vi "Dashboard Main.vi"() -> ()   [LabVIEW 2013]
uses:
  <vilib>/event_ctls.llb/eventvkey.ctl
  <vilib>/Rock Robotics/WPI/Dashboard/WPI_DashboardLogging Global.vi
  <vilib>/Utility/config.llb/Write Key (String).vi
  <vilib>/Utility/config.llb/Write Key (I32).vi
  <vilib>/Utility/config.llb/NI_LVConfig.lvlib
panel:
  out "Image Message":string="Timeout in Camera Communications"
  in  "Rec Mode":enum32{"Stop", "Record", "Playback"}(radio)
  in  "Dashboard Tab":T1(tab)
  in  "Camera Settings":T2={"Frame Rate"=30, "Compression"=30, "Size"=1} {"Frame Rate" scale=1.0..30.0; "Size" items=["640x480", "320x240", "160x120"]}
  out "MotorSliders R":cluster{"MotorSlide1":dbl, "MotorSlide2":dbl} {"MotorSlide2" scale=-1.0..1.0 scale format="%#_2e"; "MotorSlide1" scale=-1.0..1.0 scale format="%#_2e"}
  out "MotorChart R":cluster{"Numeric":dbl, "Numeric":dbl}(graph)
  out "MotorSliders L":T3 {"MotorSlide4 2" scale=0.0..14.0 scale format="%#_2e"; "MotorSlide2" scale=-1.0..1.0 scale format="%#_2e"; "MotorSlide1" scale=-1.0..1.0 scale format="%#_2e"}
  out "MotorChart L":T4(graph)
  out "JS1 Z":dbl(slide) scale=-1.0..1.0 scale format="%#_2e"
  out "Joystick 1":cluster{"X":dbl, "Y":dbl}[](graph)
  out "JS Buttons 1":T5
  out "JS2 Z":dbl(slide) scale=-1.0..1.0 scale format="%#_2e"
  out "Joystick 2":cluster{"X":dbl, "Y":dbl}[](graph)
  out "JS Buttons 2":T5
  out "Mode":T6(ring)=enum."Auto Disabled"
  out "Camera IP":string
  in  "DB Camera Config":bool
  out "fps":dbl format="%#.1g"
  out "Mbps":dbl format="%#.1g"
  out "Mbps 2":bool
  out "LED 1":bool
  in  "Slider 1":dbl(slide) scale=0.0..100.0
  in  "Checkbox 2":bool
  in  "Checkbox 1":bool
  in  "Swag Drive":bool
  out "PID":dbl=3.125
  in  "Set Pot":dbl=3.125
  in  "Smart Shooter":bool=TRUE
  in  "Power Saver":bool=TRUE
  out "Robot Code Version":string
  out "Climber Position":string
  out "Pot Voltage":dbl
  out "Shooter Speed":dbl
  in  "Test Slider":dbl(slide) scale=0.0..100.0 scale format="%#_3g"
  in  "On/Off":bool caption="Solenoid"
  in  "Test Name":u16(ring) items=["Select the test to run...", "Example Test", "-------------------------------", "List of tests is built in robot code.", "Replace with your own automated tests."]
  in  "Test Tree":string(tree)
  in  "Motor":cluster{"Value":dbl, "Enable":bool} {"Value" scale=-1.0..1.0 scale format="%#_3g"}
  out "Progress":T7 {"Test Progress" scale=0.0..100.0}
  in  "Rev/Fwd":cluster{"Forward":bool, "Reverse":bool}
  in  "Test Ring":u16(ring) items=["Auto", "Fixed indoor", "Fixed outdoor 1", "Fixed outdoor 2", "Fixed fluorescent 1", "Fixed fluorescent 2", "Hold current"]
  in  "Listbox":i32(listbox)
  out "Tree":string(tree)
  out "Camera Image":T8(plugin-control)
  in  "Enable":bool
  # "Left"
  # "Front"
  # "Right"
  # "Battery"
  # "Customize by placing controls and indicators here and name to\nmatch Dashboard Variables on robot."
  # "This tab is a great place for autonomous settings and validation.\nCustomize by placing controls and indicators here and name to\nmatch Dashboard Variables on robot."
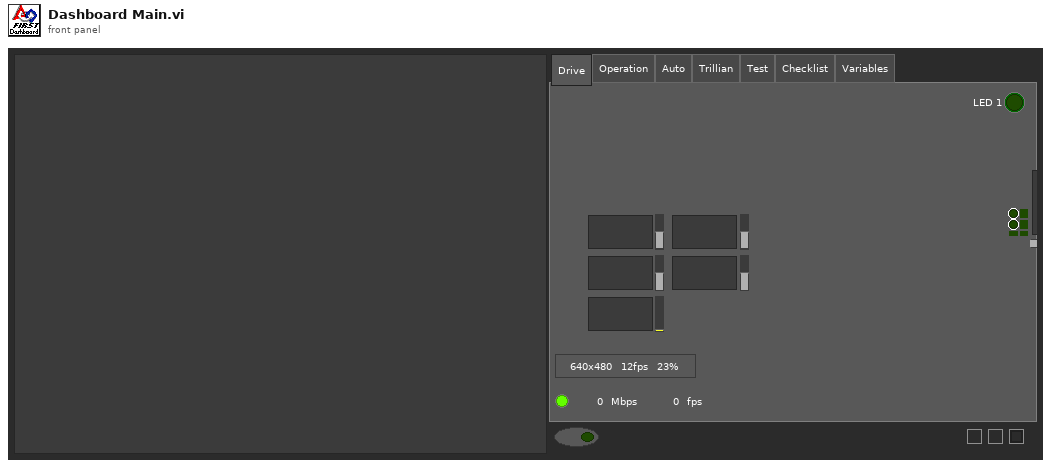
[diagram p1: front panel]
types:
  T1 = enum32{"Drive", "Operation", "Auto", "Trillian", "Test", "Checklist", "Variables"}
  T2 = cluster{"Frame Rate":i32, "Compression":i32, "Size":u16}
  T3 = cluster{"MotorSlide1":dbl, "MotorSlide2":dbl, "MotorSlide4 2":dbl}
  T4 = cluster{"Numeric":dbl, "Numeric":dbl, "Battery":sgl}
  T5 = cluster{bool, bool, bool, bool, bool, bool, bool, bool, bool, bool, bool, bool}
  T6 = enum8{"Tele-Op Disabled", "Tele-Op Enabled", "Auto Disabled", "Auto Enabled", "Test Disabled", "Test Enabled", ""}
  T7 = cluster{"Test Progress":u8, "Test Progress Text":string}
  T8 = typedef "IMAQ Image.ctl" = refnum<image>
  T9 = enum32{"Drive", "Operation", "Auto", "Test", "Checklist", "Variables"}
  T10 = typedef "Image Type" = u32
  T11 = cluster{"Digital Inputs":bool[], "Digital Outputs":bool[]}
  T12 = cluster{"Competition mode":bool, "Robot Link":bool, "Autonomous":bool, "Enabled":bool, "E-Stop":bool, "Simulated":bool, "TestMode":bool, "Docked Window":bool}
  T13 = cluster{"Boolean Array[0]":bool, "Boolean Array[1]":bool, "Boolean Array[2]":bool, "Boolean Array[3]":bool, "Boolean Array[4]":bool, "Boolean Array[5]":bool, "Boolean Array[6]":bool, "Boolean Array[7]":bool, "Boolean Array[8]":bool, "Boolean Array[9]":bool, "Boolean Array[10]":bool, "Boolean Array[11]":bool}
  T14 = typedef "NI_LVConfig.lvlib/Config Data RefNum.ctl" = refnum<k1>
  T15 = typedef "eventvkey.ctl" = enum16{"ASCII", "Enter", "Return", "Shift", "Ctrl", "Alt", "Cmd", "Opt", "Caps", "NumLock", "Clear", "Break", "Up", "Down", "Left", "Right", "Insert", "Delete", "Home", "End", "PageUp", "PageDown", "Escape", "Help", "Pause", "ScrollLock", "F1", "F2", "F3", "F4", "F5", "F6", "F7", "F8", "F9", "F10", "F11", "F12", "F13", "F14", "F15", "F16", "F17", "F18", "F19", "F20", "F21", "F22", "F23", "F24", "Play", "VolumeUp", "VolumeDown", "Mute", "Two Byte Char"}
  T16 = cluster{"Image Size":bool, "Image Type":bool, "Pixel Value":bool, "ROI Information":bool, "Zoom Factor":bool}
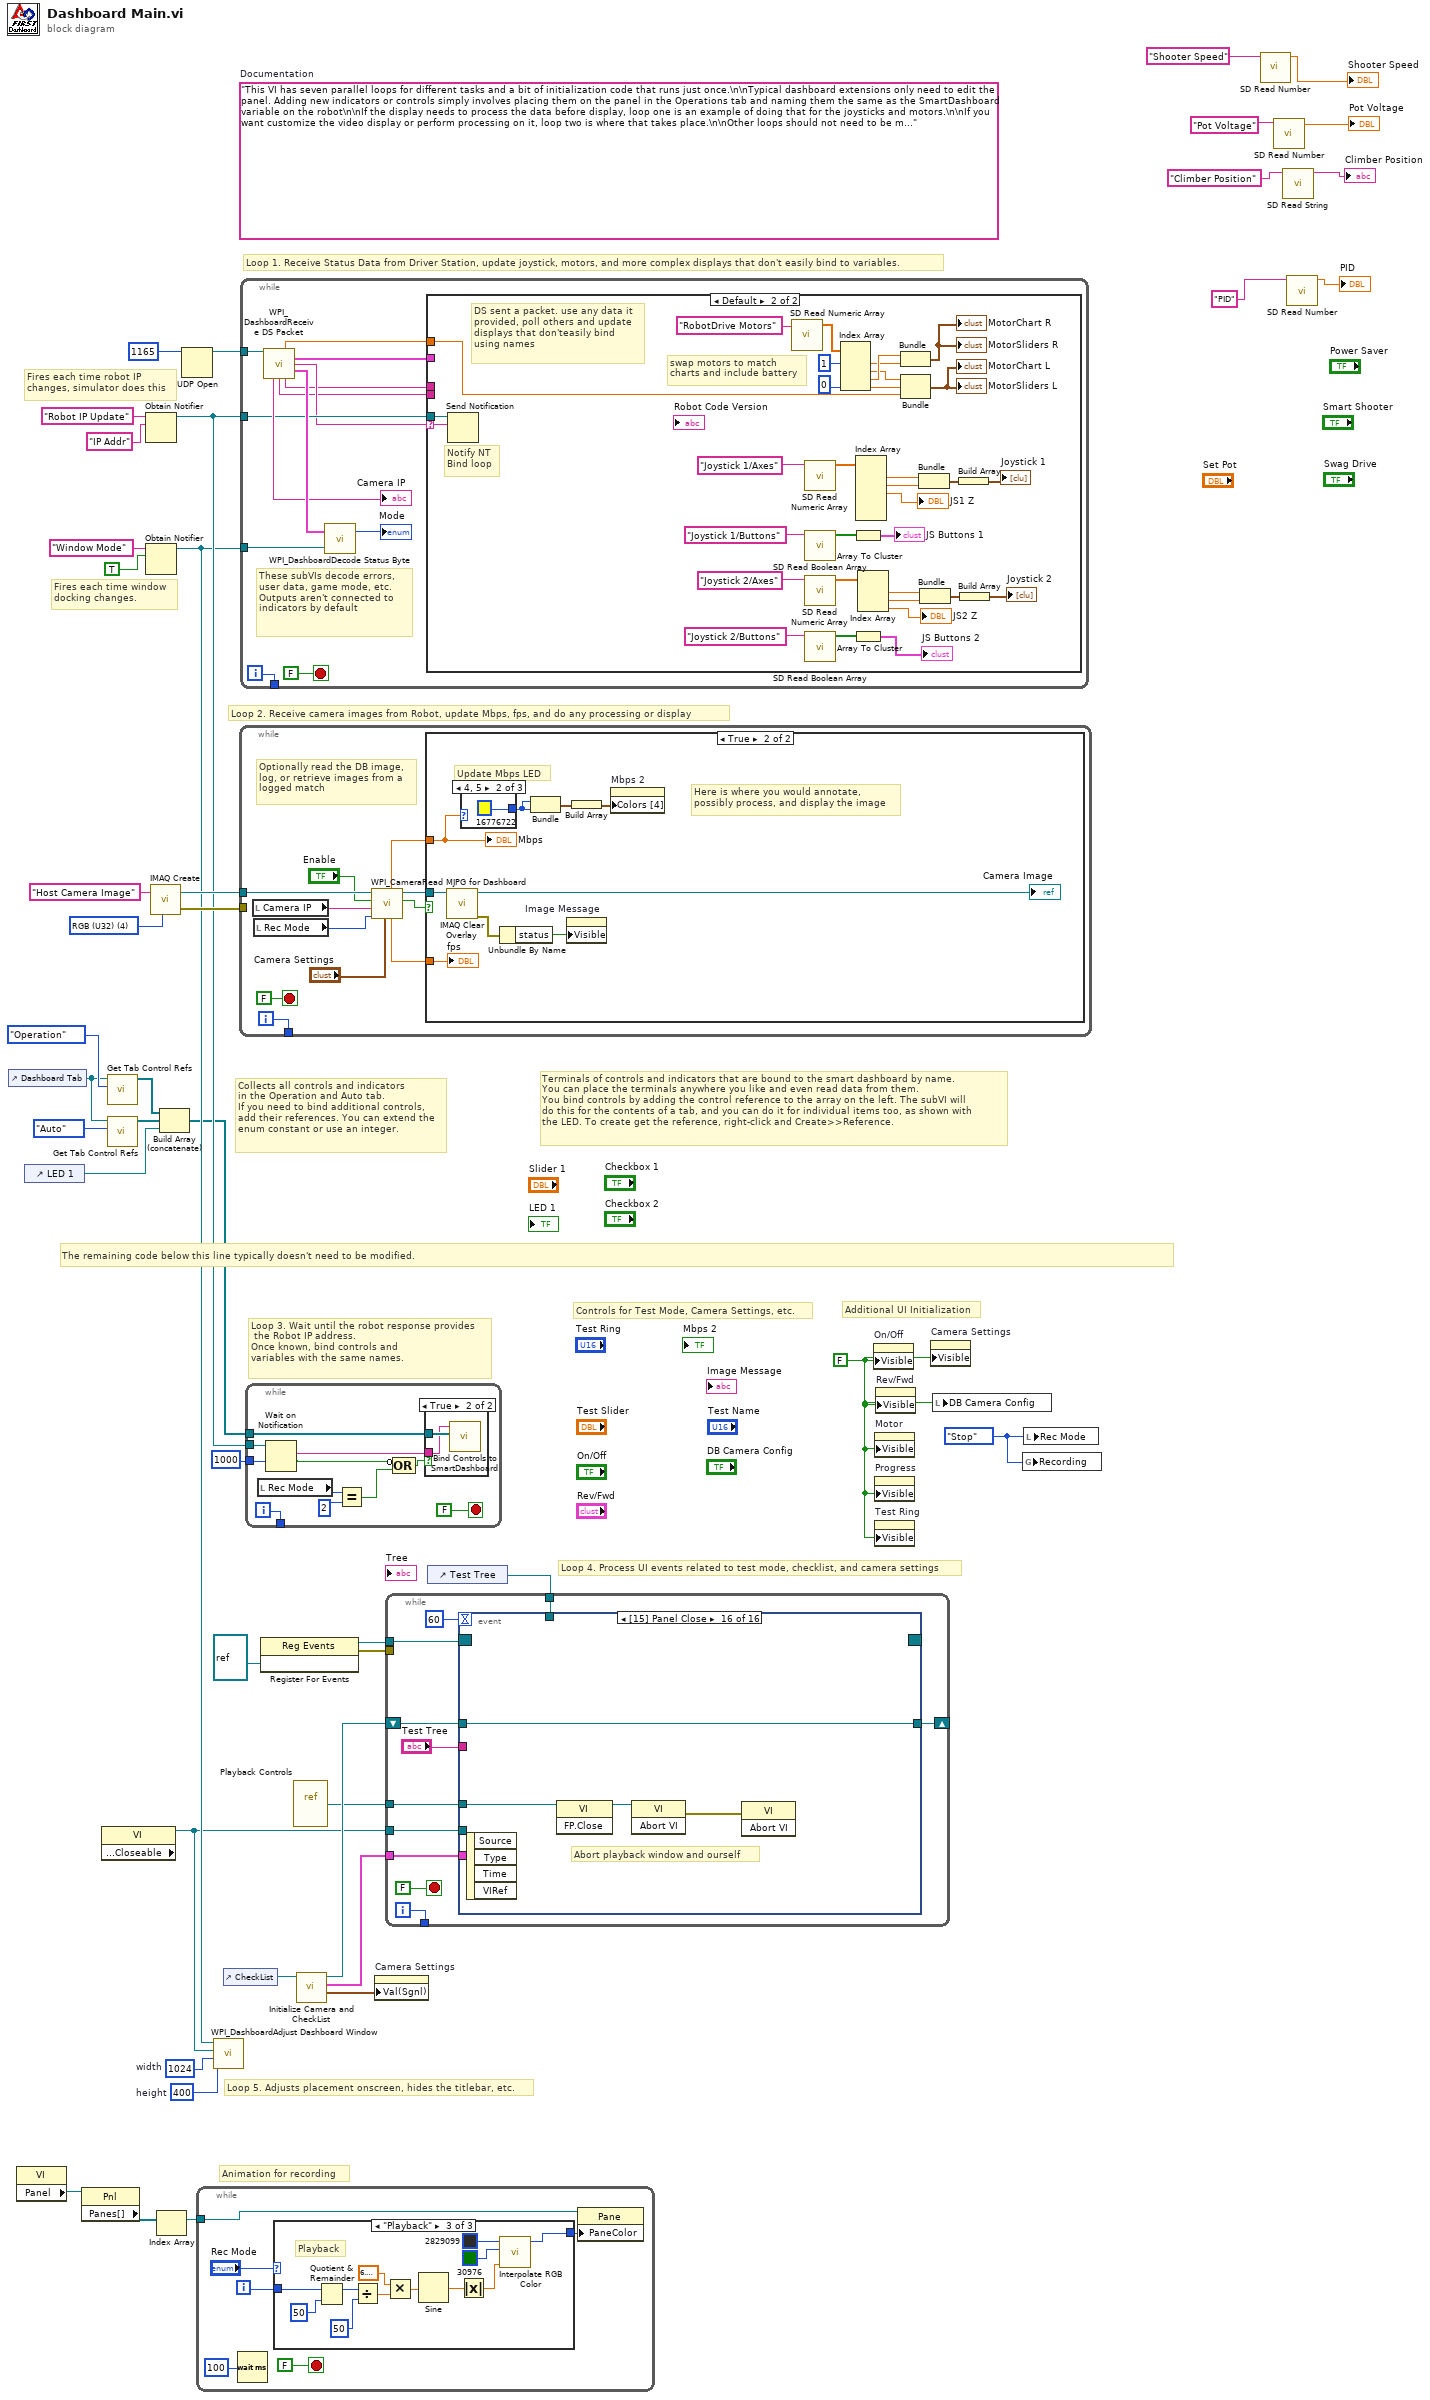
[diagram p0: block diagram]
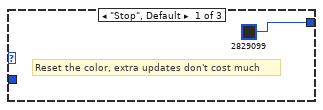
[diagram p2: hidden frame]
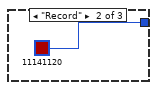
[diagram p3: hidden frame]
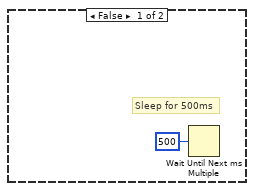
[diagram p5: hidden frame]
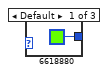
[diagram p6: hidden frame]
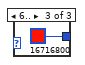
[diagram p7: hidden frame]
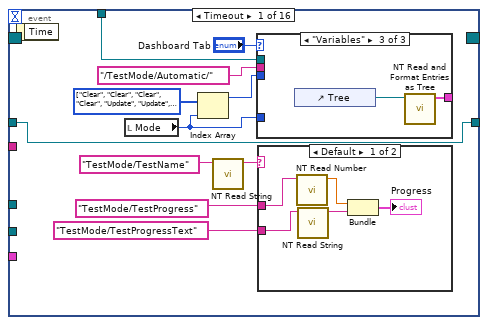
[diagram p8: hidden frame]
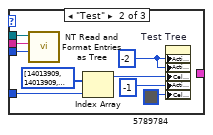
[diagram p10: hidden frame]
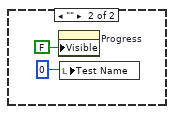
[diagram p11: hidden frame]
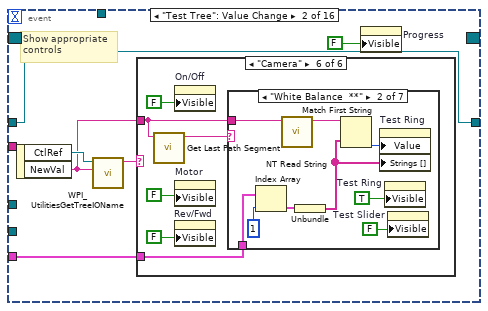
[diagram p12: hidden frame]
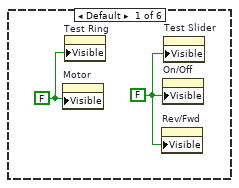
[diagram p13: hidden frame]
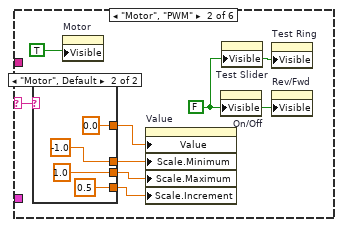
[diagram p14: hidden frame]
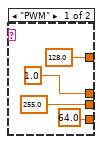
[diagram p15: hidden frame]
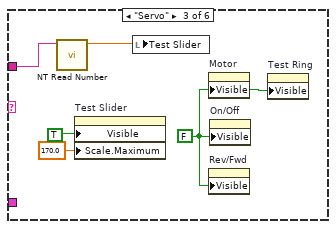
[diagram p16: hidden frame]
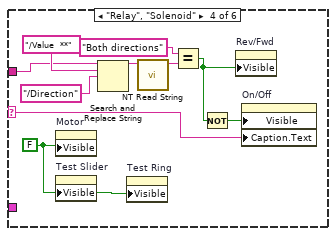
[diagram p17: hidden frame]
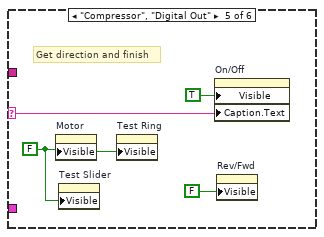
[diagram p18: hidden frame]
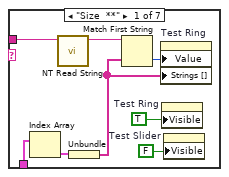
[diagram p19: hidden frame]
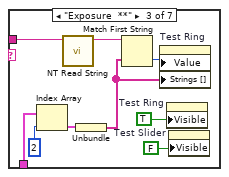
[diagram p20: hidden frame]
diagram:
  w16 = enum32{"Stop", "Record", "Playback"}."Stop" ("Rec Mode")
  w19 = 400  # height
  w20 = 1024  # width
  w33 = FALSE ("Visible")
  (unwired) "This VI has seven parallel loops for different tasks and a bit of initialization code that runs just once.\n\nTypical dashboard extensions only need to edit the panel. Adding new indicators or controls simply involves placing them on the panel in the Operations tab and naming them the same as the SmartDashboard variable on the robot\n\nIf the display needs to process the data before display, loop one is an example of doing that for the joysticks and motors.\n\nIf you want customize the video display or perform processing on it, loop two is where that takes place.\n\nOther loops should not need to be modified. They are pretty standard, and document the task they perform."  # Documentation
  w43 = T10 4 items=["Grayscale (U8)", "Grayscale (I16)", "Grayscale (SGL)", "Complex (CSG)", "RGB (U32)", "HSL (U32)", "RGB (U64)"] ("Image Type")
  # "Controls for Test Mode, Camera Settings, etc."
  # "Additional UI Initialization"
  # "Animation for recording"
  # "Fires each time robot IP\nchanges, simulator does this"
  # "Fires each time window\ndocking changes."
  # "Collects all controls and indicators\nin the Operation and Auto tab.\nIf you need to bind additional controls,\nadd their references. You can extend the\nenum constant or use an integer."
  # "The remaining code below this line typically doesn't need to be modified."
  # "Loop 4. Process UI events related to test mode, checklist, and camera settings"
  # "Terminals of controls and indicators that are bound to the smart dashboard by name.\nYou can place the terminals anywhere you like and even read data from them.\nYou bind controls by adding the control reference to the array on the left. The subVI will\ndo this for the contents of a tab, and you can do it for individual items too, as shown with\nthe LED. To create get the reference, right-click and Create>>Reference."
  # "Loop 3. Wait until the robot response provides\n the Robot IP address.\nOnce known, bind controls and\nvariables with the same names."
  # "Loop 5. Adjusts placement onscreen, hides the titlebar, etc."
  # "Loop 1. Receive Status Data from Driver Station, update joystick, motors, and more complex displays that don't easily bind to variables."
  # "Loop 2. Receive camera images from Robot, update Mbps, fps, and do any processing or display"
  n1 = control-ref of="Dashboard Tab"() -> (w14:refnum<vi>)
  n2 = property class="VI"() -> ("Panel"=w27:refnum<vi>)  [unwired: 2 in, 2 out]
  n3 = control-ref of="LED 1"() -> (w9:refnum<vi>)
  n4 = property class="Pnl"(reference=w27) -> ("Panes[]"=w28:refnum<vi>[])  [unwired: 1 in, 2 out]
  n5 = property class="VI" props=["Front Panel.Closeable"]() -> (reference out=w15:refnum<vi>)  [unwired: 2 in, 2 out]
  n6 = call <vilib>:"Get Tab Control Refs.vi"("Page Index"=T9."Operation" ("Dashboard Tab"), "TabControl in"=w14) -> ("ControlsOnPage"=w12:refnum<vi>[])  [unwired: 9 in]
  n7 = call <vilib>:"Get Tab Control Refs.vi"("Page Index"=T9."Auto" ("Dashboard Tab"), "TabControl in"=w14) -> ("ControlsOnPage"=w13:refnum<vi>[])  [unwired: 9 in]
  n8 = Obtain Notifier(name (unnamed)="Robot IP Update", notification data type="IP Addr" ("name (unnamed)")) -> (notifier out=w37:refnum<notifier>)  [unwired: 2 in, 2 out]
  n9 = Obtain Notifier(name (unnamed)="Window Mode", notification data type=TRUE) -> (notifier out=w18:refnum<notifier>)  [unwired: 2 in, 2 out]
  n10 = call "IMAQ Create"("Image Name"="Host Camera Image", "Image Type"=w43) -> ("New Image"=w41:T8, "error out"=w40:errorcluster)  [unwired: 2 in, 1 out]
  n11 = Index Array(array=w28) -> (element=w26:refnum<vi>)  [unwired: 1 in]
  n12 = Build Array (concatenate)(w12, w13, w9) -> (w11:refnum<vi>[])
  n13 = UDP Open(11:u16 1165 ("port")) -> (port=w44:refnum<k16>)  [unwired: 2 in, 4 out]
  n14 = while {
    tunnel: w26 -> [w47]
    i -> [w50]
    stop <- FALSE stop-if-true
    n15 = Wait (ms)(milliseconds to wait=u32 100) -> ()  [unwired: 1 out]
    n16 = case shown="\"Playback\"" "Rec Mode" {
      tunnel: w50 -> [_ _ w65]
      tunnel: [u32 2829099 ("Base Color") u32 11141120 ("Target Color") w54] -> w46
      frame "Stop", Default {
        # "Reset the color, extra updates don't cost much"
      }
      frame "Record" {
      }
      frame "Playback" {
        # "Playback"
        n17 = Quotient & Remainder(x=w65, y=u32 50 ("milliseconds to wait")) -> (x-y*floor(x/y)=w61:u32)  [unwired: 1 out]
        n18 = Divide(x=w61, y=u32 50 ("milliseconds to wait")) -> (x/y=w58:dbl)
        n19 = Multiply(x=6.283185307179586, y=w58) -> (x*y=w63:dbl)
        n20 = Sine(x=w63) -> (sin(x)=w62:dbl)
        n21 = Absolute Value(x=w62) -> (abs(x)=w55:dbl)
        n22 = call "Interpolate RGB Color.vi"("Proportion"=w55, "Target Color"=u32 30976, "Base Color"=u32 2829099) -> ("Result Color"=w54:u32)  [unwired: 8 in]
      }
    }
    n23 = property class="Pane"(reference=w47, "PaneColor"=w46) -> ()  [unwired: 1 in, 2 out]
  }
  n24 = call <vilib>:"WPI_DashboardAdjust Dashboard Window.vi"("height"=w19, "width"=w20, "reference in"=w15, "Notifier in"=w18) -> ()  [unwired: 8 in]
  n25 = control-ref of="CheckList"() -> (w17:refnum<vi>)
  n26 = while {
    tunnel: w41 -> [w74]
    tunnel: w40 -> [_]
    tunnel: [w75] -> _
    i -> [w75]
    stop <- FALSE stop-if-true
    # "Optionally read the DB image,\nlog, or retrieve images from a\nlogged match"
    n27 = local read "Camera IP"() -> (w67:string)
    n28 = local read "Rec Mode"() -> (w66:enum32{"Stop", "Record", "Playback"})
    n29 = call <vilib>:"WPI_CameraRead MJPG for Dashboard.vi"("Camera Settings"="Camera Settings", "Rec Mode"=w66, "Camera IP"=w67, "Enable"="Enable", "Refnum in"=w74) -> ("Active"=w71:bool, "Refnum out"=w73:T8, "FPS"=w70:dbl, "Bandwidth (Mbps)"=w69:dbl)  [unwired: 3 in]
    n30 = case shown="True" w71 {
      tunnel: w73 -> [_ w81]
      tunnel: w69 -> [_ w80]
      tunnel: w70 -> [_ w78]
      frame False {
        # "Sleep for 500ms"
        n31 = Wait Until Next ms Multiple(millisecond multiple=u32 500) -> ()  [unwired: 1 out]
      }
      frame True {
        # "Here is where you would annotate,\npossibly process, and display the image"
        # "Update Mbps LED"
        n32 = call "IMAQ Clear Overlay"("Image"=w81) -> ("error out"=w85:errorcluster, "Image Out"=→"Camera Image":T8)  [unwired: 2 in, 7 out]
        n33 = case shown="4, 5" w80 {
          tunnel: [u32 6618880 ("Color Box") u32 16776722 ("Color Box") u32 16716800 ("Color Box")] -> w82
          frame Default {
          }
          frame 4, 5 {
          }
          frame 6.. {
          }
        }
        n34 = Unbundle By Name(w85) -> ("status"=w86:bool)
        n35 = Bundle("Color Box"=w82, "Color Box"=w82) -> (w84:cluster{"Color Box":u32, "Color Box":u32})  [unwired: 1 out]
        n36 = property on="Image Message" class="Str"("Visible"=w86) -> ()  [unwired: 2 in, 2 out]
        n37 = Build Array(w84) -> (w83:cluster{"Color Box":u32, "Color Box":u32}[])
        n38 = property on="Mbps 2" class="Bool (strict)"("Colors [4]"=w83) -> ()  [unwired: 2 in, 2 out]
        "Mbps" <- w80
        "fps" <- w78
      }
    }
  }
  n39 = while {
    tunnel: w44 -> [w100]
    tunnel: w37 -> [w95]
    tunnel: w18 -> [w99]
    tunnel: [w96] -> _
    i -> [w96]
    stop <- FALSE stop-if-true
    # "These subVIs decode errors, user data, game mode, etc.\nOutputs aren't connected to indicators by default"
    n40 = call <vilib>:"WPI_DashboardReceive DS Packet.vi"("Recv Socket"=w100) -> ("Battery"=w90:sgl, "Driver Station"=w91:T11, "Robot IP Address"=w94:string, "Status"=w101:T12, "Camera IP Address"=→"Camera IP":string, "Low Priority User Data"=w93:string, "High Priority User Data"=w92:string)  [unwired: 1 in, 7 out]
    n41 = call <vilib>:"WPI_DashboardDecode Status Byte.vi"("Window Mode Notifier"=w99, "Status"=w101) -> ("Mode"=→"Mode":T6)  [unwired: 1 out]
    n42 = case shown="Default" w94 {
      selector: w94 -> [_ w113]
      tunnel: w95 -> [_ w114]
      tunnel: w93 -> [_ _]
      tunnel: w92 -> [_ _]
      tunnel: w91 -> [_ _]
      tunnel: w90 -> [_ w112]
      frame "0.0.0.0" {
        # "DS not sending packets, or no robot exists yet.\nDon't poll the variables"
      }
      frame Default {
        # "Notify NT\nBind loop"
        # "DS sent a packet. use any data it\nprovided, poll others and update\ndisplays that don'teasily bind\nusing names"
        # "swap motors to match\ncharts and include battery"
        n43 = Send Notification(notification=w113, notifier=w114) -> ()  [unwired: 1 in, 2 out]
        n44 = call <vilib>:"SD Read Numeric Array.vi"("Name"="RobotDrive Motors") -> ("Numeric Array"=w111:dbl[])  [unwired: 8 in, 2 out]
        n45 = call <vilib>:"SD Read Numeric Array.vi"("Name"="Joystick 1/Axes") -> ("Numeric Array"=w130:dbl[])  [unwired: 8 in, 2 out]
        n46 = call <vilib>:"SD Read Boolean Array.vi"("Name"="Joystick 1/Buttons") -> ("Boolean Array"=w132:bool[])  [unwired: 8 in, 2 out]
        n47 = call <vilib>:"SD Read Numeric Array.vi"("Name"="Joystick 2/Axes") -> ("Numeric Array"=w124:dbl[])  [unwired: 8 in, 2 out]
        n48 = call <vilib>:"SD Read Boolean Array.vi"("Name"="Joystick 2/Buttons") -> ("Boolean Array"=w123:bool[])  [unwired: 8 in, 2 out]
        n49 = Index Array(array=w111, index #1=1, index #4=0) -> (element #1=w107:dbl, element #2=w106:dbl, element #3=w108:dbl, element #4=w103:dbl)  [unwired: 2 in]
        n50 = Array To Cluster(array=w132) -> (cluster=→"JS Buttons 1":T13)
        n51 = Array To Cluster(array=w123) -> (cluster=→"JS Buttons 2":T13)
        n52 = Index Array(array=w130) -> (element #1=w127:dbl, element #2=w128:dbl, element #3=→"JS1 Z":dbl)  [unwired: 6 in, 3 out]
        n53 = Index Array(array=w124) -> (element #1=w119:dbl, element #2=w118:dbl, element #3=→"JS2 Z":dbl)  [unwired: 3 in]
        n54 = Bundle("Numeric"=w108, "Numeric"=w107) -> (→"MotorChart R" →"MotorSliders R":cluster{"Numeric":dbl, "Numeric":dbl})  [unwired: 1 in]
        n55 = Bundle("Numeric"=w106, "Numeric"=w103, "Battery"=w112) -> (→"MotorChart L" →"MotorSliders L":T4)  [unwired: 1 in]
        n56 = Bundle("Numeric"=w127, "Numeric"=w128) -> (w126:cluster{"Numeric":dbl, "Numeric":dbl})  [unwired: 1 in]
        n57 = Bundle("Numeric"=w119, "Numeric"=w118) -> (w120:cluster{"Numeric":dbl, "Numeric":dbl})  [unwired: 1 in]
        n58 = Build Array(w126) -> (→"Joystick 1":cluster{"Numeric":dbl, "Numeric":dbl}[])
        n59 = Build Array(w120) -> (→"Joystick 2":cluster{"Numeric":dbl, "Numeric":dbl}[])
      }
    }
  }
  n60 = while {
    tunnel: w11 -> [w146]
    tunnel: w37 -> [w144]
    tunnel: [w142] -> _
    tunnel: u32 1000 ("milliseconds to wait") -> [w141]
    i -> [w142]
    stop <- FALSE stop-if-true
    n61 = local read "Rec Mode"() -> (w137:enum32{"Stop", "Record", "Playback"})
    n62 = Wait on Notification(notifier=w144, timeout in ms (-1)=w141) -> (notification=w143:string, timed out?=w139:bool)  [unwired: 2 in, 2 out]
    n63 = Equal?(x=w137, y=u16 2 ("Rec Mode")) -> (x = y?=w138:bool)
    n64 = Compound Arithmetic op=OR(invert w139, w138) -> (w140:bool)
    n65 = case shown="True" w140 {
      tunnel: w146 -> [_ w148]
      tunnel: w143 -> [_ w147]
      frame False {
      }
      frame True {
        n66 = call <vilib>:"Bind Controls to SmartDashboard.vi"("Bound Control Refs"=w148, "Server IP Address"=w147) -> ()  [unwired: 10 in]
      }
    }
  }
  n67 = register-events(refnum<vi> refnum) -> (reference out=w24:refnum<event-registration>, error out=w23:errorcluster)  [unwired: 2 in]
  n68 = vi-ref "Playback Controls.vi"() -> (w25:refnum<vi>)
  n69 = call "Initialize Camera and CheckList.vi"("ListBox in"=w17) -> ("Cluster"=w31:cluster{"value":i32, "value":i32, "index":i32}, "Array"=w32:cluster{string[]}[], "File Refnum"=w30:T14)  [unwired: 8 in]
  n70 = property on="Camera Settings" class="Clust (strict)"("Val(Sgnl)"=w31) -> ()  [unwired: 2 in, 2 out]
  n71 = control-ref of="Test Tree"() -> (w29:refnum<vi>)
  n72 = while {
    tunnel: w32 -> [w156]
    shift-right: [w155] -> _
    shift-left: w30 -> [w154]
    tunnel: [w153] -> _
    tunnel: w29 -> [w152]
    tunnel: w25 -> [w151]
    tunnel: w24 -> [w150]
    tunnel: w23 -> [_]
    tunnel: w15 -> [w149]
    i -> [w153]
    stop <- FALSE stop-if-true
    n73 = event shown="[15] Panel Close" {
      selector: w150 -> [_ _ _ _ _ _ _ _ _ _ _ _ _ _ _ _]
      dyn-events: [_ _ _ _ _ _ _ _ _ _ _ _ _ w394 _ _] -> _
      timeout: u32 60 ("milliseconds to wait") -> [_ _ _ _ _ _ _ _ _ _ _ _ _ _ _ _]
      tunnel: w152 -> [w166 _ _ _ _ _ _ _ _ _ _ _ _ _ _ _]
      tunnel: "Test Tree" -> [_ _ _ _ _ _ _ _ w363 w371 w373 w377 w385 _ _ _]
      tunnel: w156 -> [_ w190 _ _ _ _ w327 w357 _ _ _ _ _ _ _ _]
      tunnel: [w160 w189 w288 w293 w301 w313 w326 w350 w362 w369 w372 w376 w384 w396 w410 w411] -> w155
      tunnel: w154 -> [w160 w189 w288 w293 w301 w313 w325 w350 w362 w369 w372 w376 w384 w396 w410 w411]
      tunnel: w151 -> [_ _ _ _ _ _ _ _ _ _ _ _ _ w397 _ w414]
      tunnel: w149 -> [_ _ _ _ _ _ _ _ _ _ _ _ _ w392 _ _]
      event Timeout {
        w165 = enum16{"Update", "Clear"}[] [enum."Clear", enum."Clear", enum."Clear", enum."Clear", enum."Update", enum."Update", enum."Clear"] items=["Update", "Clear"]
        n74 = event-data() -> ()  [unwired: 1 in, 1 out]
        n75 = local read "Mode"() -> (w163:T6)
        n76 = Index Array(array=w165, index=w163) -> (element=w164:enum16{"Update", "Clear"})
        n77 = call <vilib>:"NT Read String.vi"("Name"="TestMode/TestName") -> ("String"=w169:string)  [unwired: 9 in, 1 out]
        n78 = case shown="\"Variables\"" "Dashboard Tab" {
          tunnel: w166 -> [_ w179 _]
          tunnel: "/TestMode/Automatic/" ("Name Pattern") -> [_ w178 _]
          tunnel: w164 -> [_ w177 _]
          tunnel: w163 -> [_ w175 _]
          tunnel: [_ _ w181] -> _
          frame "Operation", Default {
          }
          frame "Test" {
            w174 = -2 ("Active Item:Row Number")
            n79 = call <vilib>:"NT Read and Format Entries as Tree.vi"("Operation"=w177, "Name Pattern"=w178, "Tree Refnum"=w179) -> ()  [unwired: 7 in, 2 out]
            n80 = Index Array(array=u32[] [14013909, 14013909, 14013909, 14013909, 14013909, 16777215, 14013909], index=w175) -> (element=w173:u32)
            n81 = property on="Test Tree" class="Tree (strict)"("Active Item Row Number"=w174, "ActiveColNum"=w174, "CellBG"=w173, "Active Item Row Number"=-1 ("Active Item:Row Number"), "CellBG"=u32 5789784 ("Color Box")) -> ()  [unwired: 2 in, 2 out]
          }
          frame "Variables" {
            n82 = control-ref of="Tree"() -> (w180:refnum<vi>)
            n83 = call <vilib>:"NT Read and Format Entries as Tree.vi"("Tree Refnum"=w180) -> ("Formatted Strings"=w181:cluster{"Name":string, "Value":string}[])  [unwired: 9 in, 1 out]
          }
        }
        n84 = case shown="Default" w169 {
          tunnel: "TestMode/TestProgress" ("Name") -> [w183 _]
          tunnel: "TestMode/TestProgressText" ("Name") -> [w182 _]
          frame Default {
            n85 = call <vilib>:"NT Read Number.vi"("Name"=w183) -> ("Numeric"=w184:dbl)  [unwired: 9 in, 1 out]
            n86 = call <vilib>:"NT Read String.vi"("Name"=w182) -> ("String"=w185:string)  [unwired: 9 in, 1 out]
            n87 = Bundle("Numeric"=w184, "String"=w185) -> (→"Progress":cluster{"Numeric":dbl, "String":string})  [unwired: 1 in]
          }
          frame "" {
            n88 = property on="Progress" class="Clust (strict)"("Visible"=FALSE) -> ()  [unwired: 2 in, 2 out]
            n89 = local write "Test Name"(u16 0) -> ()
          }
        }
      }
      event "Test Tree": Value Change {
        # "Show appropriate\ncontrols"
        n90 = event-data() -> ("CtlRef"=w193:refnum<vi>, "NewVal"=w191:string)  [unwired: 1 in]
        n91 = call <vilib>:"WPI_UtilitiesGetTreeIOName.vi"("NewVal"=w191, "TreeControl in"=w193) -> ("I/O Name"=w194:string)  [unwired: 9 in]
        n92 = case shown="\"Camera\"" w194 {
          selector: w194 -> [_ w201 _ w219 w228 _]
          tunnel: w191 -> [_ _ w216 w218 _ w235]
          tunnel: w190 -> [_ _ _ _ _ w234]
          frame Default {
            w196 = FALSE ("Visible")
            w195 = FALSE ("Visible")
            n93 = property on="Motor" class="Clust (strict)"("Visible"=w195) -> ()  [unwired: 2 in, 2 out]
            n94 = property on="Test Ring" class="Ring (strict)"("Visible"=w195) -> ()  [unwired: 2 in, 2 out]
            n95 = property on="Rev/Fwd" class="Clust (strict)"("Visible"=w196) -> ()  [unwired: 2 in, 2 out]
            n96 = property on="On/Off" class="Bool (strict)"("Visible"=w196) -> ()  [unwired: 2 in, 2 out]
            n97 = property on="Test Slider" class="Slide (strict)"("Visible"=w196) -> ()  [unwired: 2 in, 2 out]
          }
          frame "Motor", "PWM" {
            w202 = FALSE ("Visible")
            n98 = case shown="\"Motor\", Default" w201 {
              tunnel: [1.0 ("Value") -1.0 ("Value")] -> w200
              tunnel: [255.0 ("Value") 1.0 ("Value")] -> w199
              tunnel: [128.0 ("Value") 0.0 ("Value")] -> w198
              tunnel: [64.0 ("Value") 0.5 ("Value")] -> w197
              frame "PWM" {
              }
              frame "Motor", Default {
              }
            }
            n99 = property on="Motor" class="Clust (strict)"("Visible"=TRUE) -> ()  [unwired: 2 in, 2 out]
            n100 = property on="Value" class="Slide (strict)"("Value"=w198, "Scale.Minimum"=w200, "Scale.Maximum"=w199, "Scale.Increment"=w197) -> ()  [unwired: 2 in, 2 out]
            n101 = property on="On/Off" class="Bool (strict)"("Visible"=w202) -> ()  [unwired: 2 in, 2 out]
            n102 = property on="Test Slider" class="Slide (strict)"("Visible"=w202) -> ()  [unwired: 2 in, 2 out]
            n103 = property on="Test Ring" class="Ring (strict)"("Visible"=w202) -> ()  [unwired: 2 in, 2 out]
            n104 = property on="Rev/Fwd" class="Clust (strict)"("Visible"=w202) -> ()  [unwired: 2 in, 2 out]
          }
          frame "Servo" {
            w214 = FALSE ("Visible")
            n105 = call <vilib>:"NT Read Number.vi"("Name"=w216) -> ("Numeric"=w215:dbl)  [unwired: 9 in, 1 out]
            n106 = property on="Test Slider" class="Slide (strict)"("Visible"=TRUE, "Scale.Maximum"=170.0 ("Scale.Range:Maximum")) -> ()  [unwired: 2 in, 2 out]
            n107 = local write "Test Slider"(w215) -> ()
            n108 = property on="Motor" class="Clust (strict)"("Visible"=w214) -> ()  [unwired: 2 in, 2 out]
            n109 = property on="Rev/Fwd" class="Clust (strict)"("Visible"=w214) -> ()  [unwired: 2 in, 2 out]
            n110 = property on="On/Off" class="Bool (strict)"("Visible"=w214) -> ()  [unwired: 2 in, 2 out]
            n111 = property on="Test Ring" class="Ring (strict)"("Visible"=w214) -> ()  [unwired: 2 in, 2 out]
          }
          frame "Relay", "Solenoid" {
            w217 = FALSE ("Visible")
            n112 = property on="Motor" class="Clust (strict)"("Visible"=w217) -> ()  [unwired: 2 in, 2 out]
            n113 = property on="Test Slider" class="Slide (strict)"("Visible"=w217) -> ()  [unwired: 2 in, 2 out]
            n114 = Search and Replace String(input string=w218, search string="/Value  **", replace string="/Direction") -> (result string=w224:string)  [unwired: 5 in, 3 out]
            n115 = property on="Test Ring" class="Ring (strict)"("Visible"=w217) -> ()  [unwired: 2 in, 2 out]
            n116 = call <vilib>:"NT Read String.vi"("Name"=w224) -> ("String"=w222:string)  [unwired: 9 in, 1 out]
            n117 = Equal?(x="Both directions", y=w222) -> (x = y?=w220:bool)
            n118 = Not(x=w220) -> (.not. x?=w221:bool)
            n119 = property on="Rev/Fwd" class="Clust (strict)"("Visible"=w220) -> ()  [unwired: 2 in, 2 out]
            n120 = property on="On/Off" class="Bool (strict)"("Visible"=w221, "Caption.Text"=w219) -> ()  [unwired: 2 in, 2 out]
          }
          frame "Compressor", "Digital Out" {
            w227 = FALSE ("Visible")
            # "Get direction and finish"
            n121 = property on="Motor" class="Clust (strict)"("Visible"=w227) -> ()  [unwired: 2 in, 2 out]
            n122 = property on="Test Slider" class="Slide (strict)"("Visible"=w227) -> ()  [unwired: 2 in, 2 out]
            n123 = property on="Test Ring" class="Ring (strict)"("Visible"=w227) -> ()  [unwired: 2 in, 2 out]
            n124 = property on="On/Off" class="Bool (strict)"("Visible"=TRUE, "Caption.Text"=w228) -> ()  [unwired: 2 in, 2 out]
            n125 = property on="Rev/Fwd" class="Clust (strict)"("Visible"=FALSE) -> ()  [unwired: 2 in, 2 out]
          }
          frame "Camera" {
            n126 = call <vilib>:"Get Last Path Segment.vi"("String in"=w235) -> ("String out"=w236:string)  [unwired: 10 in]
            n127 = property on="On/Off" class="Bool (strict)"("Visible"=FALSE) -> ()  [unwired: 2 in, 2 out]
            n128 = property on="Motor" class="Clust (strict)"("Visible"=FALSE) -> ()  [unwired: 2 in, 2 out]
            n129 = property on="Rev/Fwd" class="Clust (strict)"("Visible"=FALSE) -> ()  [unwired: 2 in, 2 out]
            n130 = case shown="\"White Balance  **\"" w236 {
              tunnel: w235 -> [w242 w251 w260 w269 w278 _ w284]
              tunnel: w234 -> [w240 w248 w257 w266 w275 _ _]
              frame "Size  **" {
                n131 = Index Array(array=w240) -> (element=w239:cluster{string[]})  [unwired: 1 in]
                n132 = call <vilib>:"NT Read String.vi"("Name"=w242) -> ("String"=w241:string)  [unwired: 9 in, 1 out]
                n133 = Unbundle(w239) -> (w237:string[])
                n134 = Match First String(2:w237, 3:w241) -> (0:w238:i32)  [unwired: 1 out]
                n135 = property on="Test Ring" class="Ring (strict)"("Value"=w238, "Strings []"=w237) -> ()  [unwired: 2 in, 2 out]
                n136 = property on="Test Ring" class="Ring (strict)"("Visible"=TRUE) -> ()  [unwired: 2 in, 2 out]
                n137 = property on="Test Slider" class="Slide (strict)"("Visible"=FALSE) -> ()  [unwired: 2 in, 2 out]
              }
              frame "White Balance  **" {
                n138 = Index Array(array=w248, index=1) -> (element=w249:cluster{string[]})
                n139 = call <vilib>:"NT Read String.vi"("Name"=w251) -> ("String"=w250:string)  [unwired: 9 in, 1 out]
                n140 = Unbundle(w249) -> (w246:string[])
                n141 = Match First String(2:w246, 3:w250) -> (0:w245:i32)  [unwired: 1 out]
                n142 = property on="Test Ring" class="Ring (strict)"("Value"=w245, "Strings []"=w246) -> ()  [unwired: 2 in, 2 out]
                n143 = property on="Test Ring" class="Ring (strict)"("Visible"=TRUE) -> ()  [unwired: 2 in, 2 out]
                n144 = property on="Test Slider" class="Slide (strict)"("Visible"=FALSE) -> ()  [unwired: 2 in, 2 out]
              }
              frame "Exposure  **" {
                n145 = Index Array(array=w257, index=2) -> (element=w258:cluster{string[]})
                n146 = call <vilib>:"NT Read String.vi"("Name"=w260) -> ("String"=w259:string)  [unwired: 9 in, 1 out]
                n147 = Unbundle(w258) -> (w254:string[])
                n148 = Match First String(2:w254, 3:w259) -> (0:w255:i32)  [unwired: 1 out]
                n149 = property on="Test Ring" class="Ring (strict)"("Value"=w255, "Strings []"=w254) -> ()  [unwired: 2 in, 2 out]
                n150 = property on="Test Ring" class="Ring (strict)"("Visible"=TRUE) -> ()  [unwired: 2 in, 2 out]
                n151 = property on="Test Slider" class="Slide (strict)"("Visible"=FALSE) -> ()  [unwired: 2 in, 2 out]
              }
              frame "Exposure Priority  **" {
                n152 = Index Array(array=w266, index=3) -> (element=w267:cluster{string[]})
                n153 = call <vilib>:"NT Read String.vi"("Name"=w269) -> ("String"=w268:string)  [unwired: 9 in, 1 out]
                n154 = Unbundle(w267) -> (w263:string[])
                n155 = Match First String(2:w263, 3:w268) -> (0:w264:i32)  [unwired: 1 out]
                n156 = property on="Test Ring" class="Ring (strict)"("Value"=w264, "Strings []"=w263) -> ()  [unwired: 2 in, 2 out]
                n157 = property on="Test Ring" class="Ring (strict)"("Visible"=TRUE) -> ()  [unwired: 2 in, 2 out]
                n158 = property on="Test Slider" class="Slide (strict)"("Visible"=FALSE) -> ()  [unwired: 2 in, 2 out]
              }
              frame "Color Enable  **" {
                n159 = Index Array(array=w275, index=4) -> (element=w276:cluster{string[]})
                n160 = call <vilib>:"NT Read String.vi"("Name"=w278) -> ("String"=w277:string)  [unwired: 9 in, 1 out]
                n161 = Unbundle(w276) -> (w272:string[])
                n162 = Match First String(2:w272, 3:w277) -> (0:w273:i32)  [unwired: 1 out]
                n163 = property on="Test Ring" class="Ring (strict)"("Value"=w273, "Strings []"=w272) -> ()  [unwired: 2 in, 2 out]
                n164 = property on="Test Ring" class="Ring (strict)"("Visible"=TRUE) -> ()  [unwired: 2 in, 2 out]
                n165 = property on="Test Slider" class="Slide (strict)"("Visible"=FALSE) -> ()  [unwired: 2 in, 2 out]
              }
              frame Default {
                n166 = property on="Test Ring" class="Ring (strict)"("Visible"=FALSE) -> ()  [unwired: 2 in, 2 out]
                n167 = property on="Test Slider" class="Slide (strict)"("Visible"=FALSE) -> ()  [unwired: 2 in, 2 out]
              }
              frame "Brightness  **", "Color Level  **", "Compression  **", "FPS  **", "Sharpness  **" {
                n168 = call <vilib>:"NT Read Number.vi"("Name"=w284) -> ("Numeric"=w283:dbl)  [unwired: 9 in, 1 out]
                n169 = local write "Test Slider"(w283) -> ()
                n170 = property on="Test Slider" class="Slide (strict)"("Visible"=TRUE, "Scale.Maximum"=100.0 ("Scale.Range:Maximum")) -> ()  [unwired: 2 in, 2 out]
                n171 = property on="Test Ring" class="Ring (strict)"("Visible"=FALSE) -> ()  [unwired: 2 in, 2 out]
              }
            }
          }
        }
        n172 = property on="Progress" class="Clust (strict)"("Visible"=FALSE) -> ()  [unwired: 2 in, 2 out]
      }
      event "Test Name": Mouse Enter {
        # "Populate the ring with the list of tests"
        n173 = event-data() -> ()  [unwired: 1 in, 1 out]
        n174 = call <vilib>:"NT Read String Array.vi"("Name"="TestMode/TestList") -> ("String Array"=w292:string[])  [unwired: 9 in, 1 out]
        n175 = Build Array (concatenate)("Select the test to run...", w292) -> (w291:string[])
        n176 = property on="Test Name" class="Ring (strict)"("Strings []"=w291) -> ()  [unwired: 2 in, 2 out]
      }
      event "Test Name": Value Change {
        w294 = FALSE ("Visible")
        # "Tell the robot the test name to run"
        n177 = event-data() -> ("NewVal"=w298:u16)  [unwired: 1 in]
        n178 = property on="Test Name" class="Ring (strict)"() -> ("Strings []"=w299:string[])  [unwired: 2 in, 2 out]
        n179 = local write "Progress"(T7 {"Test Progress"=0, "Test Progress Text"=""} ("Progress")) -> ()
        n180 = Index Array(array=w299, index=w298) -> (element=w297:string)
        n181 = call <vilib>:"NT Write String.vi"("String"=w297, "Name"="TestMode/TestName") -> ()  [unwired: 9 in, 1 out]
        n182 = property on="Progress" class="Clust (strict)"("Visible"=TRUE) -> ()  [unwired: 2 in, 2 out]
        n183 = property on="Motor" class="Clust (strict)"("Visible"=w294) -> ()  [unwired: 2 in, 2 out]
        n184 = property on="Test Slider" class="Slide (strict)"("Visible"=w294) -> ()  [unwired: 2 in, 2 out]
        n185 = property on="On/Off" class="Bool (strict)"("Visible"=w294) -> ()  [unwired: 2 in, 2 out]
        n186 = property on="Rev/Fwd" class="Clust (strict)"("Visible"=w294) -> ()  [unwired: 2 in, 2 out]
        n187 = property on="Test Ring" class="Ring (strict)"("Visible"=w294) -> ()  [unwired: 2 in, 2 out]
      }
      event "Listbox": Double Click {
        n188 = event-data() -> ("PlatMods.Shift"=w302:bool, "Row"=w304:i32)  [unwired: 1 in]
        n189 = case shown="True" w302 {
          tunnel: w304 -> [w308 _]
          tunnel: 1 -> [w307 _]
          frame False {
            n190 = property on="Listbox" class="LstBox (strict)"() -> ("Item Symbols"=w306:i32[])  [unwired: 2 in, 2 out]
            n191 = Replace Array Subset(array=w306, new element=w307, index=w308) -> (w305:i32[])
            n192 = property on="Listbox" class="LstBox (strict)"("Item Symbols"=w305) -> ()  [unwired: 2 in, 2 out]
          }
          frame True {
            w309 = 0 ("Top Row")
            n193 = property on="Listbox" class="LstBox (strict)"() -> ("Number of Rows"=w311:u32)  [unwired: 2 in, 2 out]
            n194 = Initialize Array(0, w311) -> (w310:i32[])
            n195 = property on="Listbox" class="LstBox (strict)"("Top Row"=w309, "Value"=w309, "Item Symbols"=w310) -> ()  [unwired: 2 in, 2 out]
          }
        }
      }
      event "Listbox": Key Down {
        n196 = event-data() -> ("VKey"=w315:T15)  [unwired: 1 in]
        n197 = case shown="\"Left\", \"Right\"" w315 {
          selector: w315 -> [w320 _]
          tunnel: eventvkey."Left" ("VKey") -> [w318 _]
          frame "Left", "Right" {
            n198 = Equal?(x=w318, y=w320) -> (x = y?=w319:bool)
            n199 = Select(t=0, s=w319, f=1) -> (s? t:f=w321:i32)
            n200 = property on="Listbox" class="LstBox (strict)"() -> ("Item Symbols"=w324:i32[])  [unwired: 2 in, 2 out]
            n201 = Replace Array Subset(array=w324, new element=w321, index="Listbox") -> (w323:i32[])
            n202 = property on="Listbox" class="LstBox (strict)"("Item Symbols"=w323) -> ()  [unwired: 2 in, 2 out]
          }
          frame Default {
          }
        }
      }
      event "DB Camera Config": Value Change {
        n203 = event-data() -> ("NewVal"=w328:bool)  [unwired: 1 in]
        n204 = case shown="False" w328 {
          tunnel: w327 -> [w337 _]
          tunnel: [w330 w348] -> w326
          tunnel: w325 -> [w329 w348]
          frame False {
            w344 = "Camera"
            w347 = FALSE ("Visible")
            n205 = local read "Camera Settings"() -> (w336:T2)
            n206 = Index Array(array=w337) -> (element=w340:cluster{string[]})  [unwired: 1 in]
            n207 = Unbundle(w336) -> ("Frame Rate"=w335:i32, "Compression"=w334:i32, "Size"=w338:u16)
            n208 = Unbundle(w340) -> (w339:string[])
            n209 = Index Array(array=w339, index=w338) -> (element=w333:string)
            n210 = call-poly <vilib>:"Write Key.vi"("section"=w344, "value"=w333, "key"="Size", "refnum"=w329) -> ("refnum out"=w346:T14)  [unwired: 2 in, 5 out]
            n211 = call-poly <vilib>:"Write Key.vi"("section"=w344, "value"=w335, "key"="FrameRate", "refnum"=w346) -> ("refnum out"=w345:T14)  [unwired: 1 in, 6 out]
            n212 = property on="Camera Settings" class="Clust (strict)"("Visible"=w347) -> ()  [unwired: 2 in, 2 out]
            n213 = local write "DB Camera Config"(w347) -> ()
            n214 = call-poly <vilib>:"Write Key.vi"("section"=w344, "value"=w334, "key"="Compression", "refnum"=w345) -> ("refnum out"=w331:T14)  [unwired: 1 in, 6 out]
            n215 = call <vilib>:"Close Config Data.vi"("refnum"=w331) -> ("file path"=w332:path)  [unwired: 2 in, 8 out]
            n216 = call <vilib>:"Open Config Data.vi"("configuration file path"=w332) -> ("refnum"=w330:T14)  [unwired: 8 in, 2 out]
          }
          frame True {
            n217 = property on="Camera Settings" class="Clust (strict)"("Visible"=TRUE) -> ()  [unwired: 2 in, 2 out]
          }
        }
      }
      event "Camera Settings": Value Change {
        n218 = event-data() -> ("NewVal"=w361:T2)  [unwired: 1 in]
        n219 = Index Array(array=w357) -> (element=w356:cluster{string[]})  [unwired: 1 in]
        n220 = Unbundle(w361) -> ("Frame Rate"=w352:i32, "Compression"=w351:i32, "Size"=w354:u16)
        n221 = Unbundle(w356) -> (w355:string[])
        n222 = Index Array(array=w355, index=w354) -> (element=w353:string)
        n223 = Format Into String(format string="%s   %dfps   %d%%", w353, w352, w351) -> (resulting string=w358:string)  [unwired: 2 in, 1 out]
        n224 = Build Array(w358) -> (w359:string[])
        n225 = property on="DB Camera Config" class="Bool (strict)"("Strings [4]"=w359) -> ()  [unwired: 2 in, 2 out]
      }
      event "Motor.Enable": Value Change {
        n226 = event-data() -> ("NewVal"=w367:bool)  [unwired: 1 in]
        n227 = Unbundle("Motor") -> ("Value"=w366:dbl)  [unwired: 1 out]
        n228 = Select(t=w366, s=w367, f=0.0) -> (s? t:f=w364:dbl)
        n229 = call <vilib>:"NT Write Number.vi"("Numeric"=w364, "Name"=w363) -> ()  [unwired: 9 in, 1 out]
      }
      event "Test Slider": Value Change {
        n230 = event-data() -> ("NewVal"=w370:dbl)  [unwired: 1 in]
        n231 = call <vilib>:"NT Write Number.vi"("Numeric"=w370, "Name"=w371) -> ()  [unwired: 9 in, 1 out]
      }
      event "On/Off": Value Change {
        n232 = event-data() -> ("NewVal"=w375:bool)  [unwired: 1 in]
        n233 = Boolean To (0,1)(Boolean=w375) -> (0, 1=w374:i16)
        n234 = call <vilib>:"NT Write Number.vi"("Numeric"=w374, "Name"=w373) -> ()  [unwired: 9 in, 1 out]
      }
      event "Rev/Fwd": Value Change {
        n235 = event-data() -> ("NewVal.Forward"=w383:bool, "NewVal.Reverse"=w382:bool)  [unwired: 1 in]
        n236 = Boolean To (0,1)(Boolean=w383) -> (0, 1=w379:i16)
        n237 = Boolean To (0,1)(Boolean=w382) -> (0, 1=w381:i16)
        n238 = Negate(x=w381) -> (-x=w380:i16)
        n239 = Add(x=w379, y=w380) -> (x+y=w378:i16)
        n240 = call <vilib>:"NT Write Number.vi"("Numeric"=w378, "Name"=w377) -> ()  [unwired: 9 in, 1 out]
      }
      event "Test Ring": Value Change {
        n241 = event-data() -> ("NewVal"=w387:u16)  [unwired: 1 in]
        n242 = property on="Test Ring" class="Ring (strict)"() -> ("Strings []"=w388:string[])  [unwired: 2 in, 2 out]
        n243 = Index Array(array=w388, index=w387) -> (element=w386:string)
        n244 = call <vilib>:"NT Write String.vi"("String"=w386, "Name"=w385) -> ()  [unwired: 9 in, 1 out]
      }
      event "Rec Mode": Value Change {
        # "Update globals for recording mode and path to read log from.\nClear when logging and let NetworkTables set path for vision to\nuse."
        n245 = event-data() -> ("NewVal"=w398:enum32{"Stop", "Record", "Playback"})  [unwired: 1 in]
        n246 = global write "WPI_DashboardLogging Global.vi" "Logging Filename"(path "") -> ()
        n247 = case shown="\"Stop\", \"Record\"" w398 {
          tunnel: w397 -> [_ w400 w408]
          tunnel: [_ _ w407] -> w394
          tunnel: [_ _ w406] -> _
          tunnel: w392 -> [_ _ w404]
          tunnel: cluster{i32, i32} {-250, 170} -> [_ _ w403]
          tunnel: [_ _ T16 {"Image Size"=TRUE, "Image Type"=TRUE, "Pixel Value"=TRUE, "ROI Information"=TRUE, "Zoom Factor"=FALSE} ("Image Information Shown:All Elements")] -> w390
          tunnel: [_ _ TRUE ("Zoom Factor")] -> w389
          frame Default {
          }
          frame "Stop", "Record" {
            # "Place Window too"
            n248 = invoke class="VI" method="FP.Close"(reference=w400) -> (reference out=w399:refnum<vi>)  [unwired: 2 in, 2 out]
            n249 = invoke class="VI" method="Abort VI"(reference=w399) -> ()  [unwired: 2 in, 3 out]
          }
          frame "Playback" {
            n250 = call "Open Playback Panel.vi"("Offset"=w403, "DB VI Ref"=w404, "Playback in"=w408) -> ("Playback out"=w405:refnum<vi>)  [unwired: 8 in]
            n251 = register-events(w405) -> (reference out=w407:refnum<event-registration>, error out=w406:errorcluster)  [unwired: 2 in]
          }
        }
        n252 = global write "WPI_DashboardLogging Global.vi" "Recording"(w398) -> ()
        n253 = property on="Camera Image" class="ImageControl"("Image Information Shown"=w390, "Image Information Visible"=w389) -> ()  [unwired: 2 in, 2 out]
        n254 = call <vilib>:"WPI_DashboardNT Log FieldName Cache.vi"("Operation"=enum16{"Lookup/Add", "Index", "Clear"}."Clear") -> ()  [unwired: 8 in, 3 out]
      }
      event Panel Close {
        w409 = enum32{"Stop", "Record", "Playback"}."Stop" ("Rec Mode")
        n255 = event-data() -> ()  [unwired: 1 in, 4 out]
        n256 = local write "Rec Mode"(w409) -> ()
        n257 = global write "WPI_DashboardLogging Global.vi" "Recording"(w409) -> ()
      }
      event Panel Close {
        # "Abort playback window and ourself"
        n258 = event-data() -> ()  [unwired: 1 in, 4 out]
        n259 = invoke class="VI" method="FP.Close"(reference=w414) -> (reference out=w413:refnum<vi>)  [unwired: 2 in, 2 out]
        n260 = invoke class="VI" method="Abort VI"(reference=w413) -> (error out=w412:errorcluster)  [unwired: 2 in, 2 out]
        n261 = invoke class="VI" method="Abort VI"(error in=w412) -> ()  [unwired: 2 in, 3 out]
      }
    }
  }
  n262 = property on="On/Off" class="Bool (strict)"("Visible"=w33) -> ()  [unwired: 2 in, 2 out]
  n263 = property on="Motor" class="Clust (strict)"("Visible"=w33) -> ()  [unwired: 2 in, 2 out]
  n264 = property on="Progress" class="Clust (strict)"("Visible"=w33) -> ()  [unwired: 2 in, 2 out]
  n265 = property on="Test Ring" class="Ring (strict)"("Visible"=w33) -> ()  [unwired: 2 in, 2 out]
  n266 = property on="Rev/Fwd" class="Clust (strict)"("Visible"=w33) -> ()  [unwired: 2 in, 2 out]
  n267 = property on="Camera Settings" class="Clust (strict)"("Visible"=w33) -> ()  [unwired: 2 in, 2 out]
  n268 = local write "DB Camera Config"(w33) -> ()
  n269 = global write "WPI_DashboardLogging Global.vi" "Recording"(w16) -> ()
  n270 = local write "Rec Mode"(w16) -> ()
  n271 = call <vilib>:"SD Read Number.vi"("Name"="Shooter Speed") -> ("Numeric"=→"Shooter Speed":dbl)  [unwired: 8 in, 2 out]
  n272 = call <vilib>:"SD Read Number.vi"("Name"="Pot Voltage") -> ("Numeric"=→"Pot Voltage":dbl)  [unwired: 8 in, 2 out]
  n273 = call <vilib>:"SD Read String.vi"("Name"="Climber Position") -> ("String"=→"Climber Position":string)  [unwired: 8 in, 2 out]
  n274 = call <vilib>:"SD Read Number.vi"("Name"="PID") -> ("Numeric"=→"PID":dbl)  [unwired: 8 in, 2 out]
